vi "10-Tap 8-Bit Camera with DRAM (Host) - const.vi"() -> ()   [LabVIEW 2018]
doc: "This is the host VI for the 10-Tap 8-Bit Camera with DRAM example. This example demonstrates how to acquire images from a 10-tap, 8-bit, extended configuration, Camera Link camera and display the images on the host. This example supports area scan and line scan cameras for both continuous and finite acquisitions.\n\nThis example also demonstrates the use of DRAM as a frame buffer for very high speed acquisitions. Data packing and flow-control are also employed to maximize use of the available DRAM and FIFOs in terms of both memory space and performance.\n\nAdditionally, the example demonstrates the serial server, which allows third-party camera configuration utilities to communicate with the camera using the Camera Link serial interface while this VI is running."
uses:
  <vilib>/userdefined/High Color/nirio_resource_hc.ctl
  <vilib>/Analysis/Matrix/Datatypes/RealMatrix.ctl
  <vilib>/Platform/TimedLoop/XDataNode/timing_clust.ctl
  <vilib>/Platform/TimedLoop/XDataNode/nitl_modes.ctl
  <vilib>/Platform/TimedLoop/XDataNode/wakeup.ctl
  <vilib>/DAQmx/write.llb/DAQmx Write (Analog DBL 1Chan 1Samp).vi
  <vilib>/Analysis/baseanly.llb/Real A x B.vi
  <vilib>/FPGAPlugInAG/PCIe-1473R/niLvFpga_Open_PCIe-1473R.vi
  <vilib>/rvi/interface/common/dynamic/niFpgaDynamicAddResources.vi
  <vilib>/FPGAPlugInAG/Dynamic/niLvFpga_Reset_Dynamic.vi
  <vilib>/Analysis/Matrix/Numeric/Conversions/Array To Matrix - RA2.vi
  <userlib>/DAQNavi Polymorphic VI/create/DAQNavi Create Channel(CI-UpDown Count Value).vi
  <vilib>/Utility/error.llb/Error Cluster From Error Code.vi
  <vilib>/rvi/errors/niLvFpgaAdjustHostInterfaceError.vi
  <vilib>/FPGAPlugInAG/Dynamic/niLvFpga_Run_Dynamic.vi
  <vilib>/rvi/interface/common/niFpgaWaitOnOcc.vi
  <userlib>/DAQNavi Polymorphic VI/read/DAQNavi Read (Counter Count Value 1Chan 1Samp).vi
  <vilib>/Analysis/Matrix/Numeric/Conversions/Array To Matrix - RA.vi
  <vilib>/Analysis/Matrix/Numeric/Conversions/Matrix To Array - RM.vi
  <vilib>/DAQmx/miscellaneous.llb/DAQmx Fill In Error Info.vi
  <vilib>/FPGAPlugInAG/Dynamic/niLvFpga_Close_Dynamic.vi
  <vilib>/platform/TimedLoop/XDataNode/XDataNode.xnode
  <vilib>/rvi/interface/nirviOpenFPGA/nirviOpenFPGA.xnode
  FPGA Bitfiles/10-Tap8-bitCamer_FPGATarget_10-Tap8-bitCamer_C490DC32.lvbitx
  <vilib>/rvi/interface/nirviMethod/nirviMethod.xnode
  <vilib>/ErrorRing/Error Ring.xnode
  <vilib>/rvi/interface/nirviReadWriteControl/nirviReadWriteControl.xnode
  <vilib>/rvi/interface/nirviCloseFPGA/nirviCloseFPGA.xnode
  <vilib>/rvi/interface/Simulation/niFpgaSimulationCallBeginRW.vi
  <vilib>/rvi/errors/niLvFpgaMergeErrorWithErrorCode.vi
  NiFpgaLv.dll
  <vilib>/FPGAPlugInAG/Dynamic/niLvFpga_ConfigureFifo_Dynamic.vi
  <vilib>/FPGAPlugInAG/Dynamic/niLvFpga_StartFifo_Dynamic.vi
  <vilib>/FPGAPlugInAG/Dynamic/niLvFpga_ReadFifo_Dynamic.vi
  <vilib>/Platform/TimedLoop/XDataNode/XDNodeRunTimeDep.lvlib
  <resource>/objmgr/ni.dex.rc
  MPC_dll_4_vs17_cv3_4/x64/Release/MPC_dll_4_vs17_cv3_4.dll
  fish tracking dll vc17 opencv3_4/x64/Release/fish tracking dll vc17 opencv3_4.dll
  <vilib>/Analysis/NI_AALBase.lvlib
  <vilib>/Analysis/Matrix/NI_Matrix.lvlib
panel:
  in  "shift":i32=9
  in  "gamma":dbl=0.015 format="%#_13g"
  out "Cluster":cluster{"data":i32, i32}
  out "Real Matrix 5":T1
  out "Real Matrix 4":T1
  out "Real Matrix 2":T1
  out "Real Matrix":T1
  out "A x B 2":T1
  out "A x B":T1
  out "error out":errorcluster
  in  "send":bool
  out "Is Connected":bool
  in  "update ratio":dbl=0.1
  in  "Start Serial Server":bool=TRUE
  in  "Stopped 2":bool
  in  "display":bool=TRUE
  out "Image":T2(plugin-control)
  in  "reset 2":bool
  in  "reset frame":bool
  in  "reset position":bool
  out "max load a frame":dbl
  out "max load a position":dbl
  out "# elements in queue":i32
  out "element":dbl[](array[numeric])
  in  "start sending":bool
  out "connected":bool
  in  "Acquire":bool
  out "max distance 2":i32
  out "out of FOV 2":i32
  in  "count":bool
  out "max distance":i32
  out "out of FOV":i32
  out "Stage Position Y":i32=520
  out "Stage Position X":i32=520
  out "#timeout3":i32
  out "#timeout1":i32
  out "max time4 image and position loading":dbl
  out "max time3 total":dbl
  out "max time2 detection":dbl
  out "max time1 detection+command":dbl
  out "time loading a frame":dbl
  in  "length of fish_history":i32=4
  in  "m(length of kernel)":i32=30
  out "Heading":cluster{dbl, dbl}
  out "BKG_Global":T2(plugin-control)
  out "process":i32
  in  "Target Y":i32(slide)=171 min=0 max=384 scale=130.0..230.0
  in  "Target X":i32(slide)=179 min=0 max=520 scale=130.0..230.0
  out "y":dbl
  out "x":dbl
  in  "Controller":picture
  out "Y Resolution":i32
  out "X Resolution":i32
  in  "Track":bool
  out "Frame #":i32=72
  out "电压2":dbl
  out "电压1":dbl
  out "fish FOUND":bool
  out "Centroid":cluster{"x":i32, "y":i32}
  out "TimeDelay":dbl
  in  "DMA Buffer Size\n(In Images)":u32=64 caption="DMA Buffer Size"
  in  "Signal Mapping":T3(ring)=enum."Basler 10-tap"
  out "Acq In Progress":bool
  in  "Line Scan":bool
  in  "Cancel":bool
  out "Acq'd Frame Width":u32
  in  "Stopped":bool
  in  "RIO Device":T4="RIO0"
  out "DMA Write Timeout":bool
  out "Frames Acq'd":u32
  out "Acq'd Frame Height":u32
  in  "Stop":bool
  in  "Image Height":u32=360 max=65535
  in  "Image Width":u32=360 max=65535 step=40
  out "Initialized":bool
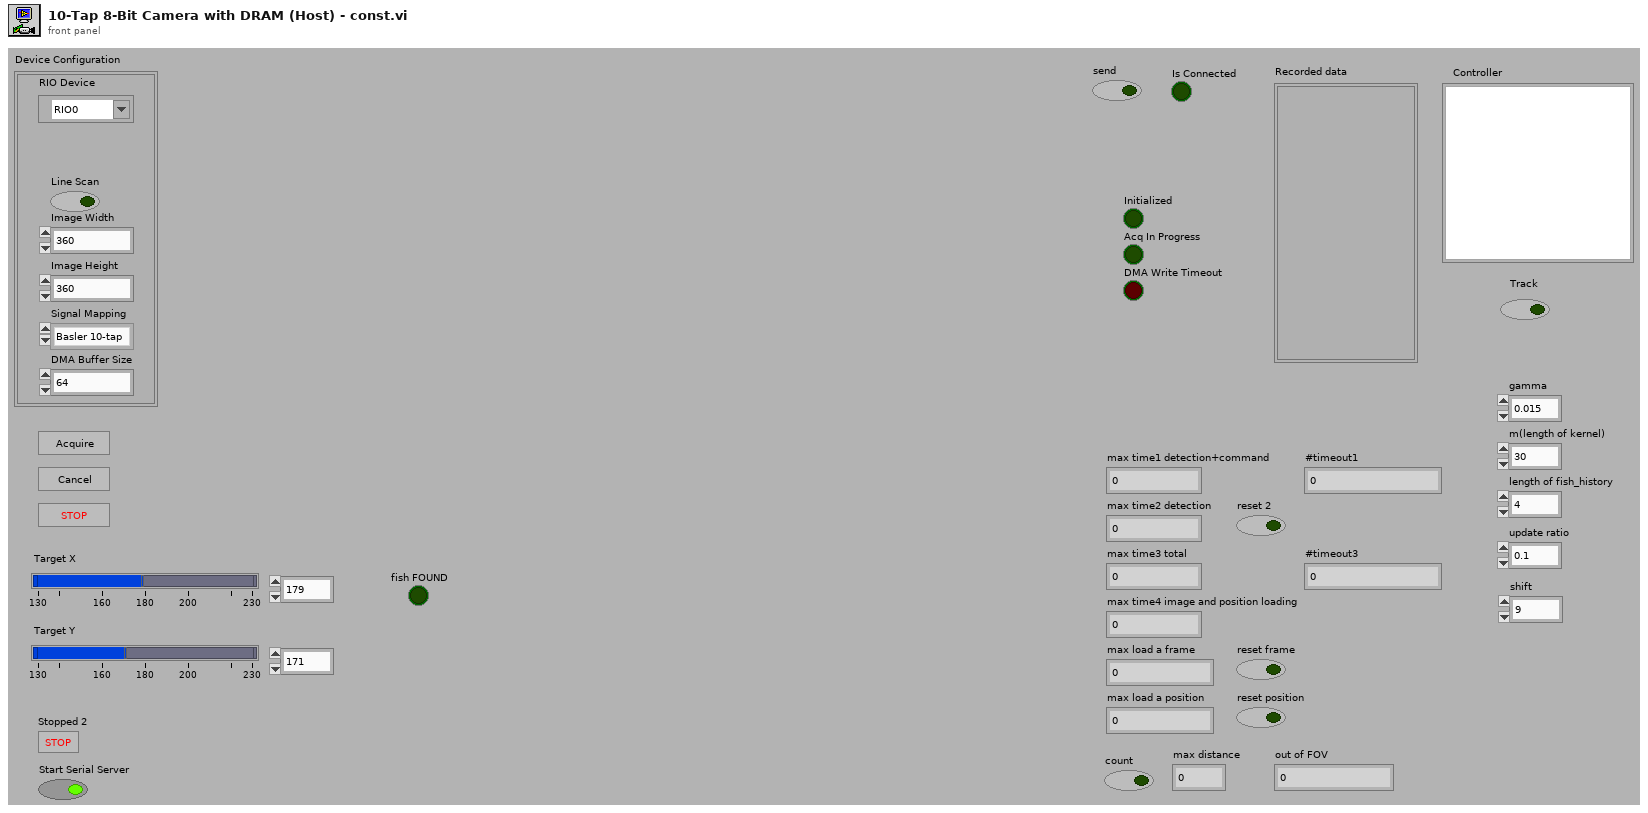
[diagram p1: front panel]
types:
  T1 = typedef "NI_Matrix.lvlib/RealMatrix.ctl" = dbl[][]
  T2 = typedef "IMAQ Image.ctl" = refnum<image>
  T3 = enum8{"Standard", "Basler 10-tap", "Vosskühler 10-tap"}
  T4 = typedef "nirio_resource_hc.ctl" = tag
  T5 = typedef "Image Type" = u32
  T6 = typedef "XDNodeRunTimeDep.lvlib/timing_clust.ctl" = cluster{"Expected End [f-1]":u64, "Actual End [f-1]":u64, "Finished Late? [f-1]":bool, "Expected End [i-1]":u64, "Actual End [i-1]":u64, "Finished Late? [i-1]":bool, "Expected Start [i]":u64, "Actual Start [i]":u64, "Expected Start [f]":u64, "Actual Start [f]":u64, "Source Name":string, "Structure Name":string, "Period":i64, "Deadline":i64, "Offset":i64, "Start":i64, "Priority":i32, "Timeout":i32, "Mode":T7, "Wakeup Reason":T8, "Error":errorcluster, "Source Type":string, "Secondary Source Type":string, "Global End Time":u64, "Global Start Time":u64, "Frame Duration":u64, "Iteration Duration":u64, "Assigned CPU":i32, "I/O Scan Engine Mode":u32}
  T7 = typedef "XDNodeRunTimeDep.lvlib/nitl_modes.ctl" = enum32{"No Change", "Process missed periods, maintain original phase", "Discard missed periods, maintain original phase", "Process missed periods, ignore original phase", "Discard missed periods, ignore original phase"}
  T8 = typedef "XDNodeRunTimeDep.lvlib/wakeup.ctl" = enum32{"Normal", "Aborted", "Asynchronous wakeup", "Timing source error", "Timed loop error", "Timeout"}
  T9 = enum16{"big-endian, network order", "native, host order", "little-endian"}
  T10 = enum32{"Map Pixel Pointer", "Unmap Pixel Pointer", "Get Pixels Infos"}
  T11 = typedef "LVPoint32TypeDef.ctl" = cluster{"Horizontal":i32, "Vertical":i32}
  T12 = typedef "LVPositionTypeDef.ctl" = cluster{"Left":i32, "Top":i32}
  T13 = typedef "LVBoundsTypeDef.ctl" = cluster{"Width":u32, "Height":u32}
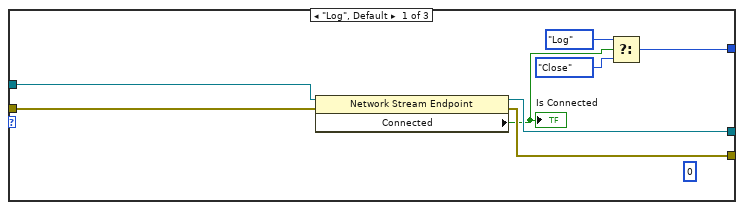
[diagram p4: hidden frame]
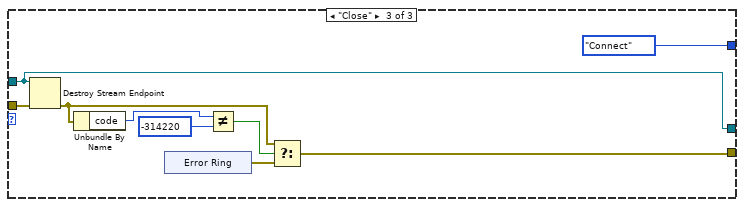
[diagram p5: hidden frame]
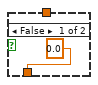
[diagram p12: hidden frame]
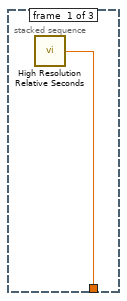
[diagram p13: hidden frame]
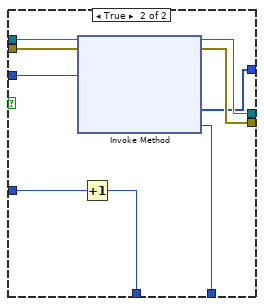
[diagram p14: hidden frame]
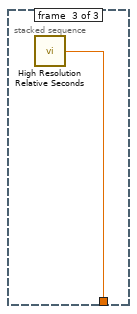
[diagram p15: hidden frame]
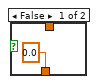
[diagram p16: hidden frame]
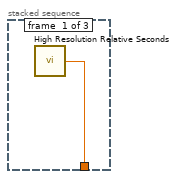
[diagram p17: hidden frame]
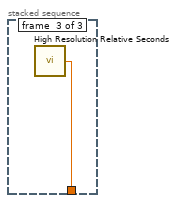
[diagram p20: hidden frame]
diagram:
  w23 = 72 ("n_templates")
  w25 = 0
  w46 = 2
  w40 = 0
  w47 = 0.0
  w72 = T5 0 items=["Grayscale (U8)", "Grayscale (I16)", "Grayscale (SGL)", "Complex (CSG)", "RGB (U32)", "HSL (U32)", "RGB (U64)", "Grayscale (U16)"] ("Image Type")
  w86 = refnum<k21> "Stage_Y"  # DAQmx任务名
  w87 = refnum<k21> "Stage_X"  # DAQmx任务名
  w89 = T5 0 items=["Grayscale (U8)", "Grayscale (I16)", "Grayscale (SGL)", "Complex (CSG)", "RGB (U32)", "HSL (U32)", "RGB (U64)", "Grayscale (U16)"] ("Image Type")
  w95 = u32 8  # Pixels per DMA word
  w126 = T5 0 items=["Grayscale (U8)", "Grayscale (I16)", "Grayscale (SGL)", "Complex (CSG)", "RGB (U32)", "HSL (U32)", "RGB (U64)", "Grayscale (U16)"] ("Image Type")
  # "Start the Serial Server to allow serial communication\nwith the camera. This allows third-party camera\nconfiguration utilites to be used."
  # "If your camera outputs active-low enable\nsignals or does not use DVAL then you \ncan change the configuration here."
  # "Configure the DMA FIFO memory buffer to be\nlarge enough for several frames. This provides\nbuffering to help deal with system latencies."
  # "Start running\nthe FPGA VI."
  # "Reset FPGA to clear\nany current state."
  # "Read the specified image\nwidth and height. In this\nexample, these must be set\nbefore starting the VI."
  # "Merge any errors.\nClean up the image.\nClose the FPGA reference.\nDisplay any errors."
  # "Acquire frames as requested.\nUse the width and height to determine how much data to read from the DMA FIFO.\nConvert the data into a Vision Image for display."
  # "Monitor the acquisition status"
  # "Create an image of the type to be displayed."
  # "Initialize the acquisition interface on the FPGA.  This will\nwait until a pixel clock is detected from the camera."
  # "Initialize the DMA FIFO for transferring\ndata from FPGA target to the host."
  # "Configure the Camera Link interface.\nThis needs to be done prior to running\nthe FPGA block diagram."
  # "Open a reference to the FPGA bitstream\nand initialize the user interface."
  n1 = flat-sequence {
    tunnel: [w132] -> w121
    tunnel: [w131] -> w130
    frame #0 {
      w135 = u32 0 ("Num Lines Acq'd")
      w134 = FALSE ("stop")
      n2 = local write "DMA Write Timeout"(w134) -> ()
      n3 = local write "Acq'd Frame Width"(w135) -> ()
      n4 = local write "Acq'd Frame Height"(w135) -> ()
      n5 = local write "Stopped"(w134) -> ()
      n6 = local write "Frames Acq'd"(w135) -> ()
      n7 = local write "Initialized"(w134) -> ()
      n8 = xnode "打开FPGA VI引用句柄"("resource name"="RIO Device") -> ("FPGA VI Reference Out"=w132:refnum<k20>, "error out"=w131:errorcluster)  [unwired: 1 in]
    }
  }
  n9 = xnode "Invoke Method"("FPGA VI Reference In"=w121, "error in"=w130) -> ("FPGA VI Reference Out"=w111:refnum<k20>, "error out"=w113:errorcluster)
  n10 = xnode "Read/Write Control"("FPGA VI Reference In"=w111, "error in"=w113, "CL Config.FVAL Active High"=TRUE ("IO Module Config.CL FVAL Active High"), "CL Config.LVAL Active High"=TRUE ("IO Module Config.CL LVAL Active High"), "CL Config.DVAL Active High"=TRUE ("IO Module Config.CL DVAL Active High"), "CL Config.Spare Active High"=TRUE ("IO Module Config.CL Spare Active High"), "CL Config.Line Scan"="Line Scan", "Acq Control.Ignore DVAL"=FALSE ("CL Config.Line Scan"), "CL Config.Configuration"=enum8{"Base", "Medium", "Full"}."Full", "CL Config.Signal Mapping"="Signal Mapping") -> ("FPGA VI Reference Out"=w114:refnum<k20>, "error out"=w112:errorcluster)
  n11 = xnode "Invoke Method"("FPGA VI Reference In"=w114, "error in"=w112) -> ("FPGA VI Reference Out"=w92:refnum<k20>, "error out"=w91:errorcluster)  [unwired: 1 in]
  n12 = Multiply(x="Image Height", y="Image Width") -> (x*y=w94:u32)
  n13 = Quotient & Remainder(x=w94, y=w95) -> (floor(x/y)=w93:u32)  [unwired: 1 out]
  n14 = Multiply(x=w93, y="DMA Buffer Size\n(In Images)") -> (x*y=w105:u32)
  n15 = xnode "Invoke Method"("FPGA VI Reference In"=w92, "error in"=w91, "请求的深度"=w105) -> ("FPGA VI Reference Out"=w120:refnum<k20>, "error out"=w119:errorcluster)  [unwired: 1 out]
  n16 = xnode "Invoke Method"("FPGA VI Reference In"=w120, "error in"=w119) -> ("FPGA VI Reference Out"=w106:refnum<k20>, "error out"=w118:errorcluster)
  n17 = xnode "读取/写入控件"("FPGA VI Reference In"=w106, "error in"=w118, "Acq Control.Initialize"=TRUE ("Arm Acquisition")) -> ("FPGA VI Reference Out"=w129:refnum<k20>, "error out"=w128:errorcluster)
  n18 = while {
    tunnel: w129 -> [w143]
    tunnel: w128 -> [w142]
    tunnel: [w141] -> w10
    tunnel: [w145] -> w102
    i -> [w137]
    stop <- w148 stop-if-true
    # "A custom error is generated if the acquisition unit has not become\ninitialized within 2 seconds. This typically occurs when a camera is\nnot connected, is not powered, or is not of the correct type."
    n19 = xnode "读取/写入控件"("FPGA VI Reference In"=w143, "error in"=w142) -> ("FPGA VI Reference Out"=w141:refnum<k20>, "error out"=w140:errorcluster, "Acq Status.Initialized"=w139:bool)
    n20 = Wait (ms)(milliseconds to wait=u32 100) -> ()  [unwired: 1 out]
    n21 = Greater?(x=w137, y=20) -> (0:w138:bool)
    n22 = case shown="True" w138 {
      tunnel: [w150 FALSE] -> w144
      tunnel: w139 -> [w150 _]
      tunnel: w140 -> [w149 w152]
      tunnel: [w149 w154] -> w145
      frame False {
      }
      frame True {
        n23 = Merge Errors(w152, errorcluster {"status"=TRUE, "code"=-8999, "source"="Acquisition Initialization: This error typically occurs when a camera is not properly connected, is not powered, or is not of the correct type."} ("error in")) -> (w154:errorcluster)
      }
    }
    "Initialized" <- w144
    n24 = Unbundle By Name(w145) -> ("status"=w147:bool)
    n25 = Or(x=w147, y=w144) -> (x .or. y?=w148:bool)
  }
  n26 = case shown="True" "Start Serial Server" {
    tunnel: [_ w155] -> w9
    tunnel: w10 -> [_ w156]
    frame False {
    }
    frame True {
      n27 = control-ref of="Stopped 2"() -> (w157:refnum<vi>)
      n28 = call "SerialServer.vi"("Stop Refnum"=w157, "FPGA VI Reference In"=w156) -> ("FPGA VI Reference Out"=w155:refnum<k20>)  [unwired: 5 in]
    }
  }
  n29 = call "IMAQ Create"("Image Name"="Image", "Image Type"=w126, "error in (no error)"=w102) -> ("New Image"=w99:T2, "error out"=w98:errorcluster)  [unwired: 2 in]
  n30 = Add(x="length of fish_history", y=1) -> (x+y=w42:i32)
  n31 = Initialize Array(0.0, 7) -> (w12:dbl[])
  n32 = Obtain Queue(max queue size (-1, unlimited)=3, name (unnamed)="tracking result" ("Image Name"), element data type=w12) -> (queue out=w8:refnum<queue>)  [unwired: 2 in, 2 out]
  n33 = Multiply(x=w46, y=w42) -> (x*y=w39:i32)
  n34 = To Unsigned Byte Integer(number=w25) -> (unsigned 8bit integer=w26:u8)
  n35 = Add(x="m(length of kernel)", y=1) -> (x+y=w27:i32)
  n36 = Initialize Array(w26, w25, w25, w25) -> (w24:u8[][][])
  n37 = for {
    N: w23 -> [_]
    shift-right: [w159] -> w22
    shift-left: w24 -> [w160]
    i -> [w158]
    w164 = T5 0 items=["Grayscale (U8)", "Grayscale (I16)", "Grayscale (SGL)", "Complex (CSG)", "RGB (U32)", "HSL (U32)", "RGB (U64)", "Grayscale (U16)"] ("Image Type")
    n38 = Number To Decimal String(number=w158) -> (decimal integer string=w168:string)  [unwired: 1 in]
    n39 = Concatenate Strings(w168, ".jpg") -> (w167:string)
    n40 = Build Path(base path=path "F:/TrackingUsingOpenCV3_with_bkg_subtr_and_pred_and_temp_matching_nodisplay - 210309/templates" ("Templates Path"), name or relative path=w167) -> (appended path=w166:path)
    n41 = call "IMAQ Create"("Image Name"="Temp", "Image Type"=w164) -> ("New Image"=w163:T2)  [unwired: 3 in, 1 out]
    n42 = call "IMAQ ReadFile"("File Path"=w166, "Image"=w163) -> ("Image Out"=w162:T2)  [unwired: 5 in, 4 out]
    n43 = call "IMAQ ImageToArray"("Image"=w162) -> ("Image Pixels (U8)"=w161:u8[][])  [unwired: 3 in, 4 out]
    n44 = Insert Into Array(array=w160, index (dim 0)=w158, new element=w161) -> (w159:u8[][][])  [unwired: 2 in]
  }
  n45 = Multiply(x=w46, y=w27) -> (x*y=w45:i32)
  n46 = Obtain Queue(max queue size (-1, unlimited)=w45, name (unnamed)="command_history", element data type=w47) -> (queue out=w49:refnum<queue>)  [unwired: 2 in, 2 out]
  n47 = Obtain Queue(max queue size (-1, unlimited)=w39, name (unnamed)="stage_position_history", element data type=w40) -> (queue out=w38:refnum<queue>)  [unwired: 2 in, 2 out]
  n48 = Obtain Queue(max queue size (-1, unlimited)=w39, name (unnamed)="fish_tr_history", element data type=w40) -> (queue out=w51:refnum<queue>)  [unwired: 2 in, 2 out]
  n49 = Obtain Queue(max queue size (-1, unlimited)=w39, name (unnamed)="fish_heading_history", element data type=w47) -> (queue out=w50:refnum<queue>)  [unwired: 2 in, 2 out]
  n50 = for "For循环" {
    N: w45 -> [_]
    tunnel: w49 -> [w173]
    tunnel: [w172] -> w48
    n51 = Lossy Enqueue Element(queue=w173, element=0.0) -> (queue out=w172:refnum<queue>)  [unwired: 1 in, 3 out]
  }
  n52 = call-poly <userlib>:"DAQNavi Create Channel.vi"("physical channels"="PCI-1784,BID#1/cntr0" ("Image Name"), "signal counting type"="AbPhaseX4" ("Image Name"), "initial value"="0" ("Image Name")) -> ("task out"=w66:i32)  [unwired: 11 in, 1 out]
  n53 = call-poly <userlib>:"DAQNavi Create Channel.vi"("physical channels"="PCI-1784,BID#1/cntr1" ("Image Name"), "signal counting type"="AbPhaseX4" ("Image Name"), "initial value"="0" ("Image Name")) -> ("task out"=w65:i32)  [unwired: 11 in, 1 out]
  n54 = call "IMAQ Create"("Image Name"="BkgImageOpenCV", "Image Type"=w72) -> ("New Image"=w74:T2)  [unwired: 3 in, 1 out]
  n55 = call <userlib>:"DAQNavi Start Task.vi"("task in"=w66) -> ("task out"=w62:i32)  [unwired: 9 in, 1 out]
  n56 = call <userlib>:"DAQNavi Start Task.vi"("task in"=w65) -> ("task out"=w61:i32)  [unwired: 9 in, 1 out]
  n57 = while "Target->Host Data Writer" {
    shift-right: [w181] -> w2
    shift-left: _ -> [w184]
    shift-right: [w180] -> _
    shift-left: _ -> [w185]
    shift-right: [w182] -> _
    shift-left: enum16{"Log", "Connect", "Close"}."Log" -> [w183]
    tunnel: w8 -> [w176]
    tunnel: [w175] -> w1
    stop <- w174 stop-if-true
    # "Send Data to Host VI"
    n58 = case shown="\"Connect\"" w183 {
      tunnel: [w202 w209 w227] -> w180
      tunnel: w185 -> [w205 _ w227]
      tunnel: w184 -> [w204 _ w228]
      tunnel: [w203 w210 w221] -> w181
      tunnel: [w206 enum16{"Log", "Connect", "Close"}."Log" enum16{"Log", "Connect", "Close"}."Connect"] -> w182
      frame "Log", Default {
        (unwired) 0 ("timeout ms")
        n59 = property class="Network Stream Endpoint"(reference=w205, error in=w204) -> (reference out=w202:refnum<k21>, error out=w203:errorcluster, "Connected"=w201:bool)
        "Is Connected" <- w201
        n60 = Select(t=enum16{"Log", "Connect", "Close"}."Log", s=w201, f=enum16{"Log", "Connect", "Close"}."Close") -> (s? t:f=w206:enum16{"Log", "Connect", "Close"})
      }
      frame "Connect" {
        n61 = Concatenate Strings("//" ("reader url"), "192.168.1.30" ("Target IP Address")) -> (w215:string)
        n62 = Concatenate Strings(w215, "/reader1" ("reader url")) -> (w213:string)
        n63 = Create Network Stream Writer Endpoint(5:-1 ("timeout in ms (-1)"), 7:70, 9:0.0, 10:w213, 11:"writer") -> (0:w210:errorcluster, 3:w209:refnum<k21>)  [unwired: 2 in]
      }
      frame "Close" {
        n64 = Destroy Stream Endpoint(8:w228, 11:w227) -> (0:w222:errorcluster)
        n65 = Unbundle By Name(w222) -> ("code"=w226:i32)
        n66 = xnode "Error Ring"() -> ("error out"=w223:errorcluster)
        n67 = Not Equal?(x=w226, y=-314220) -> (x != y?=w224:bool)
        n68 = Select(t=w222, s=w224, f=w223) -> (s? t:f=w221:errorcluster)
      }
    }
    n69 = property class="Network Stream Endpoint"(reference=w180, error in=w181) -> (reference out=w178:refnum<k21>, error out=w177:errorcluster, "Connected"=w179:bool)
    n70 = case shown="True" w179 {
      tunnel: w178 -> [_ w190]
      tunnel: w177 -> [_ w191]
      tunnel: w176 -> [w186 w189]
      tunnel: [w186 w187] -> w175
      frame False {
      }
      frame True {
        n71 = Get Queue Status(queue=w189) -> (queue out=w193:refnum<queue>)  [unwired: 2 in, 7 out]
        n72 = Dequeue Element(queue=w193) -> (queue out=w187:refnum<queue>, element=w192:dbl[])  [unwired: 2 in, 2 out]
        n73 = case shown="True" "send" {
          tunnel: w192 -> [_ w198]
          tunnel: w191 -> [_ w197]
          tunnel: w190 -> [_ w196]
          frame False {
          }
          frame True {
            w199 = 0 ("timeout ms (-1)")
            n74 = shared-variable-write(w196, w197, w198, w199) -> (w195:refnum<k21>, w200:errorcluster)  [unwired: 1 out]
            n75 = Flush Stream(8:w200, 9:w199, 11:w195) -> (0:→"error out":errorcluster)  [unwired: 1 in, 2 out]
          }
        }
      }
    }
    n76 = local read "Stop"() -> (w174:bool)
  }
  n77 = disable-structure shown="Disabled" {
    disable-tunnel: w8 -> [w231 _]
    frame Disabled {
      n78 = Concatenate Strings("//" ("reader url"), "192.168.1.19" ("Target IP Address")) -> (w242:string)
      n79 = Concatenate Strings(w242, "/reader1" ("reader url")) -> (w240:string)
      n80 = Create Network Stream Writer Endpoint(7:70, 9:0.0, 10:w240, 11:"writer") -> (0:w245:errorcluster, 3:w247:refnum<k21>)  [unwired: 3 in]
      n81 = property class="Network Stream Endpoint"(reference=w247, error in=w245) -> (reference out=w238:refnum<k21>, error out=w237:errorcluster, "Connected"=→"connected":bool)
      n82 = node-c288() -> (w251:T6)  [unwired: 4 in]
      n83 = timed-loop {
        tunnel: w231 -> [w258]
        tunnel: w238 -> [w257]
        tunnel: w237 -> [w256]
        tunnel: [w255] -> w234
        tunnel: [w254] -> w233
        tunnel: [w253] -> w232
        timing: w251 -> [_]
        timing-out: [_] -> w250
        stop <- w252 stop-if-true
        n84 = node-c288() -> ()  [unwired: 1 in, 1 out]
        n85 = case shown="True" "start sending" {
          tunnel: w257 -> [w263 w276]
          tunnel: w256 -> [w262 w275]
          tunnel: w258 -> [w264 w266]
          tunnel: [w264 w274] -> w255
          tunnel: [w263 w269] -> w254
          tunnel: [w262 w268] -> w253
          frame False {
          }
          frame True {
            w270 = 0
            n86 = Get Queue Status(queue=w266) -> (queue out=w267:refnum<queue>, # elements in queue=w265:i32)  [unwired: 2 in, 6 out]
            n87 = disable-structure shown="Disabled" {
              disable-tunnel: w265 -> [w277 _]
              frame Disabled {
                "# elements in queue" <- w277
              }
              frame Enabled {
              }
            }
            n88 = Dequeue Element(queue=w267) -> (queue out=w274:refnum<queue>, element=w273:dbl[])  [unwired: 2 in, 2 out]
            n89 = disable-structure shown="Disabled" {
              disable-tunnel: w273 -> [w278 _]
              frame Disabled {
                "element" <- w278
              }
              frame Enabled {
              }
            }
            n90 = shared-variable-write(w276, w275, w273, w270) -> (w272:refnum<k21>, w271:errorcluster)  [unwired: 1 out]
            n91 = Flush Stream(8:w271, 9:w270, 11:w272) -> (0:w268:errorcluster, 3:w269:refnum<k21>)  [unwired: 1 in, 1 out]
          }
        }
        n92 = local read "Stop"() -> (w252:bool)
        n93 = node-c288() -> ()  [unwired: 1 in, 1 out]
      }
      n94 = node-c288(w250) -> ()  [unwired: 1 out]
      n95 = Release Queue(queue=w234) -> ()  [unwired: 2 in, 3 out]
      n96 = Flush Stream(8:w232, 11:w233) -> (0:w235:errorcluster, 3:w236:refnum<k21>)  [unwired: 2 in, 1 out]
      n97 = Destroy Stream Endpoint(8:w235, 11:w236) -> ()  [unwired: 1 out]
    }
    frame Enabled {
    }
  }
  n98 = call-poly <vilib>:"Array To Matrix.vi"("Real 2D Array"=dbl[][] [[1.506559, -0.036078], [0.030048, 1.495542]]) -> ("Real Matrix"=w4:T1)
  "Real Matrix 5" <- w4
  n99 = call "IMAQ ReadFile"("File Path"=path "F:/TrackingUsingOpenCV3_with_bkg_subtr_and_pred_and_temp_matching_nodisplay/fish tracking dll vc17 opencv3_4/bkg_global.png" ("Bkg Image Path"), "Image"=w74) -> ("Image Out"=w71:T2)  [unwired: 5 in, 4 out]
  n100 = call-poly <vilib>:"Array To Matrix.vi"("Real 2D Array"=dbl[][] [[1.506559, -0.036078, 0.0], [0.030048, 1.495542, 1.506559], [-12.463135, -1.547689, 1.0]]) -> ("Real Matrix"=w5:T1)
  "Real Matrix 4" <- w5
  n101 = node-c288() -> (w17:T6)  [unwired: 4 in]
  n102 = call "IMAQ Create"("Image Name"="DstImageOpenCV", "Image Type"=w89) -> ("New Image"=w88:T2)  [unwired: 3 in, 1 out]
  n103 = while {
    tunnel: w10 -> [w291]
    tunnel: [w294] -> w115
    stop <- w293 stop-if-true
    w284 = u32 10  # Pixels per clock
    # "Update status indicators"
    n104 = Wait Until Next ms Multiple(millisecond multiple=u32 100) -> ()  [unwired: 1 out]
    n105 = xnode "Read/Write Control"("FPGA VI Reference In"=w291) -> ("error out"=w290:errorcluster, "Acq Status.Lines Per Frame"=w287:u32, "Acq Status.Frames Acq'd"=w289:u32, "Acq Status.Clocks Per Line"=w285:u32, "Acq Status.Acq In Progress"=→"Acq In Progress":bool, "Acq Status.DMA Write Timeout"=w282:bool)  [unwired: 1 in, 1 out]
    "DMA Write Timeout" <- w282
    n106 = Multiply(x=w285, y=w284) -> (x*y=w286:u32)
    n107 = disable-structure shown="Disabled" {
      disable-tunnel: w289 -> [w297 _]
      disable-tunnel: w287 -> [w296 _]
      disable-tunnel: w286 -> [w295 _]
      frame Disabled {
        "Acq'd Frame Height" <- w296
        "Frames Acq'd" <- w297
        "Acq'd Frame Width" <- w295
      }
      frame Enabled {
      }
    }
    n108 = local read "Stopped"() -> (w281:bool)
    n109 = Compound Arithmetic op=AND(w282, invert w281) -> (w283:bool)
    n110 = case shown="True" w283 {
      tunnel: w290 -> [w302 _]
      tunnel: [w302 errorcluster {"status"=TRUE, "code"=-8999, "source"="DMA Write Timeout: The write operation to the DMA FIFO on the FPGA timed out. This can be caused by the DMA FIFO not being started or the DMA FIFO overflowing. Make sure that Start is being called on the DMA FIFO. Also make sure that the host application is reading from the DMA FIFO fast enough to prevent it from overflowing."} ("error out")] -> w294
      frame False {
      }
      frame True {
      }
    }
    n111 = flat-sequence {
      tunnel: w294 -> [w301]
      tunnel: [w299] -> w293
      frame #0 {
        n112 = Unbundle By Name(w301) -> ("status"=w300:bool)
        n113 = Or(x=w300, y="Stopped") -> (x .or. y?=w299:bool)
        n114 = local write "Stopped"(w299) -> ()
      }
    }
  }
  n115 = call <vilib>:"Simple Error Handler.vi"("error in (no error)"=w2) -> ()  [unwired: 4 in, 5 out]
  n116 = Release Queue(queue=w1) -> ()  [unwired: 2 in, 3 out]
  n117 = Open/Create/Replace File(file path (use dialog)=path "E:/Time.txt" ("Folder"), operation (0:open)=4) -> (refnum out=w31:refnum<file>)  [unwired: 4 in, 2 out]
  n118 = call <vilib>:"DAQmx Start Task.vi"("task/channels in"=w86) -> ("task out"=w84:refnum<k21>)  [unwired: 13 in, 1 out]
  n119 = call <vilib>:"DAQmx Start Task.vi"("task/channels in"=w87) -> ("task out"=w85:refnum<k21>)  [unwired: 13 in, 1 out]
  n120 = timed-loop {
    tunnel: w10 -> [w427]
    tunnel: w98 -> [w426]
    tunnel: w93 -> [w323]
    tunnel: "Image Height" -> [w322]
    tunnel: "Image Width" -> [w431]
    tunnel: w99 -> [w430]
    tunnel: [w312] -> w116
    tunnel: [w429] -> w125
    tunnel: [w428] -> w123
    tunnel: w88 -> [w425]
    tunnel: w85 -> [w424]
    tunnel: w84 -> [w423]
    tunnel: [w422] -> w83
    tunnel: [w421] -> w82
    tunnel: w71 -> [w420]
    tunnel: w62 -> [w413]
    tunnel: w61 -> [w412]
    tunnel: [w411] -> w58
    tunnel: [w410] -> w57
    shift-right: [w416] -> _
    shift-left: u32 0 -> [w417]
    shift-right: [w414] -> _
    shift-left: cluster{"y":i32, "x":i32} {"y"=0, "x"=0} ("Centroid") -> [w415]
    tunnel: w48 -> [w409]
    tunnel: w51 -> [w408]
    tunnel: w50 -> [w407]
    tunnel: w38 -> [w406]
    tunnel: [w405] -> w37
    tunnel: [w404] -> w36
    tunnel: [w403] -> w35
    tunnel: [w402] -> w34
    tunnel: w31 -> [w400]
    tunnel: [w399] -> w30
    shift-right: [w398] -> _
    shift-left: _ -> [w397]
    tunnel: w23 -> [w396]
    tunnel: w22 -> [w395]
    tunnel: w8 -> [w394]
    timing: w17 -> [_]
    timing-out: [_] -> w16
    border: u32 0 -> [_]
    tunnel: w5 -> [w308]
    tunnel: w4 -> [w306]
    i -> [w401]
    stop <- w418 stop-if-true
    # "Read one frame\nfrom DMA FIFO"
    # "If we're in an acquisition, wait until\nwe have at least one frame to read."
    n121 = node-c288() -> ()  [unwired: 1 in, 1 out]
    n122 = stacked-sequence {
      tunnel: [_ w442 _] -> w429
      tunnel: w427 -> [_ w441 _]
      tunnel: w426 -> [_ w440 _]
      tunnel: [_ w439 _] -> w312
      tunnel: [_ w438 _] -> w393
      tunnel: w323 -> [_ w437 _]
      tunnel: w322 -> [_ w436 _]
      tunnel: [w435 _ _] -> w320
      tunnel: [_ _ w490] -> w321
      frame #0 {
        n123 = call <vilib>:"High Resolution Relative Seconds.vi"() -> ("relative seconds"=w435:dbl)
      }
      frame #1 {
        n124 = while {
          tunnel: [w448] -> w438
          tunnel: w437 -> [w445]
          shift-right: [w456] -> w442
          shift-left: w441 -> [w455]
          shift-right: [w449] -> w439
          shift-left: w440 -> [w454]
          tunnel: w436 -> [w443]
          stop <- w444 stop-if-true
          n125 = feedback #1() -> (w450:u32)
          n126 = while {
            tunnel: w455 -> [w486]
            tunnel: w454 -> [w485]
            tunnel: [w483] -> w453
            tunnel: [w484] -> w452
            tunnel: w450 -> [w489]
            tunnel: [w487] -> w446
            stop <- w488 stop-if-true
            n127 = xnode "Read/Write Control"("FPGA VI Reference In"=w486, "error in"=w485, "Acq Control.Cancel Acq"="Cancel") -> ("FPGA VI Reference Out"=w484:refnum<k20>, "error out"=w483:errorcluster, "Acq Status.Acq In Progress"=w482:bool, "Acq Status.Frames Acq'd"=w481:u32)
            n128 = Greater?(x=w481, y=w489) -> (0:w487:bool)
            n129 = Compound Arithmetic op=OR(invert w482, w487) -> (w488:bool)
          }
          n130 = case shown="False" w446 {
            tunnel: w445 -> [w468 w479]
            tunnel: [w463 w478] -> w456
            tunnel: w453 -> [w470 w477]
            tunnel: w452 -> [w469 w476]
            tunnel: [w457 w475] -> w451
            tunnel: w450 -> [w458 w474]
            tunnel: [w462 w473] -> w449
            tunnel: [_ w472] -> w448
            tunnel: [w468 w471] -> w447
            tunnel: w443 -> [w467 _]
            frame False {
              n131 = xnode "Read/Write Control"("FPGA VI Reference In"=w469, "error in"=w470, "Acq Control.Line Scan Height"=w467, "Acq Control.Frames To Acq"=u32 0 ("Frames To Acquire")) -> ("FPGA VI Reference Out"=w465:refnum<k20>, "error out"=w464:errorcluster)
              n132 = call "Rising Edge Detect.vi"("Input"="Acquire") -> ("Pulse"=w461:bool)  [unwired: 4 in]
              n133 = xnode "Read/Write Control"("FPGA VI Reference In"=w465, "error in"=w464, "Acq Control.Acquire"=w461) -> ("FPGA VI Reference Out"=w463:refnum<k20>, "error out"=w462:errorcluster)
              n134 = Select(t=u32 0, s="Acquire", f=w458) -> (s? t:f=w457:u32)
            }
            frame True {
              n135 = xnode "Invoke Method"("FPGA VI Reference In"=w476, "error in"=w477, "元素数量"=w479) -> ("FPGA VI Reference Out"=w478:refnum<k20>, "error out"=w473:errorcluster, "数据"=w472:u64[], "剩余元素"=w471:u32)  [unwired: 1 in]
              n136 = Increment(x=w474) -> (x+1=w475:u32)
            }
          }
          n137 = feedback-in #1(w451) -> ()
          n138 = Less?(x=w447, y=w445) -> (x < y?=w444:bool)
        }
      }
      frame #2 {
        n139 = call <vilib>:"High Resolution Relative Seconds.vi"() -> ("relative seconds"=w490:dbl)
      }
    }
    n140 = disable-structure shown="Disabled" {
      disable-tunnel: w401 -> [w432 _]
      frame Disabled {
        "process" <- w432
      }
      frame Enabled {
      }
    }
    n141 = Not(x="reset frame") -> (.not. x?=w311:bool)
    n142 = Boolean To (0,1)(Boolean=w311) -> (0, 1=w316:i16)
    n143 = Subtract(x=w321, y=w320) -> (x-y=w317:dbl)
    n144 = feedback #2(-inf) -> (w319:dbl)
    n145 = Max & Min(x=w317, y=w319) -> (max(x,y)=w314:dbl)  [unwired: 1 out]
    n146 = Multiply(x=w314, y=w316) -> (x*y=w313:dbl)
    n147 = feedback-in #2(w313) -> ()
    n148 = case shown="True" w311 {
      tunnel: w314 -> [_ w434]
      tunnel: [0.0 w434] -> w310
      frame False {
      }
      frame True {
      }
    }
    "max load a frame" <- w310
    n149 = flat-sequence {
      tunnel: w397 -> [w512]
      tunnel: w406 -> [w513]
      tunnel: w407 -> [w514]
      tunnel: w408 -> [w515]
      tunnel: w409 -> [w516]
      tunnel: w412 -> [w510]
      tunnel: w413 -> [w511]
      tunnel: w415 -> [w517]
      tunnel: w417 -> [w518]
      tunnel: w420 -> [w519]
      tunnel: w425 -> [w520]
      tunnel: w393 -> [w521]
      tunnel: w430 -> [w522]
      tunnel: w431 -> [w523]
      tunnel: w322 -> [w524]
      tunnel: [w524] -> w392
      tunnel: [w523] -> w391
      tunnel: [w522] -> w390
      tunnel: [w521] -> w389
      tunnel: [w520] -> w388
      tunnel: [w519] -> w387
      tunnel: [w518] -> w386
      tunnel: [w517] -> w385
      tunnel: [w516] -> w384
      tunnel: [w515] -> w383
      tunnel: [w514] -> w382
      tunnel: [w513] -> w381
      tunnel: [w512] -> w380
      tunnel: [w509] -> w379
      tunnel: [w508] -> w378
      tunnel: [w507] -> w377
      tunnel: [w506] -> w376
      tunnel: w396 -> [w506]
      tunnel: [w505] -> w375
      tunnel: w395 -> [w505]
      tunnel: w394 -> [w504]
      tunnel: [w504] -> w374
      tunnel: w308 -> [w492]
      tunnel: [w492] -> w307
      tunnel: w306 -> [w491]
      tunnel: [w491] -> w304
      tunnel: [w571] -> w373
      tunnel: [w570] -> w372
      tunnel: [w569] -> w371
      tunnel: [w568] -> w370
      tunnel: [w567] -> w369
      tunnel: [w566] -> w368
      tunnel: [w565] -> w367
      tunnel: [w564] -> w366
      tunnel: [w546] -> w365
      tunnel: [w544] -> w364
      tunnel: [w563] -> w363
      tunnel: [w562] -> w362
      tunnel: [w561] -> w361
      tunnel: [w560] -> w360
      tunnel: [w556] -> w359
      tunnel: [w545] -> w358
      tunnel: w392 -> [w571]
      tunnel: w391 -> [w570]
      tunnel: w390 -> [w569]
      tunnel: w389 -> [w568]
      tunnel: w388 -> [w567]
      tunnel: w387 -> [w566]
      tunnel: w386 -> [w565]
      tunnel: w385 -> [w564]
      tunnel: w384 -> [w563]
      tunnel: w383 -> [w562]
      tunnel: w382 -> [w561]
      tunnel: w381 -> [w560]
      tunnel: w380 -> [w554]
      tunnel: w379 -> [w546]
      tunnel: w378 -> [w545]
      tunnel: w377 -> [w544]
      tunnel: [w543] -> w357
      tunnel: w376 -> [w543]
      tunnel: [w542] -> w356
      tunnel: w375 -> [w542]
      tunnel: [w541] -> w355
      tunnel: w374 -> [w541]
      tunnel: [w540] -> w309
      tunnel: w307 -> [w540]
      tunnel: [w539] -> w305
      tunnel: w304 -> [w539]
      tunnel: w401 -> [w623]
      tunnel: w400 -> [w622]
      tunnel: [w621] -> w399
      tunnel: w373 -> [w672]
      tunnel: w372 -> [w671]
      tunnel: w371 -> [w670]
      tunnel: w370 -> [w668]
      tunnel: w369 -> [w597]
      tunnel: w368 -> [w643]
      tunnel: w367 -> [w640]
      tunnel: w366 -> [w595]
      tunnel: w365 -> [w616]
      tunnel: w364 -> [w615]
      tunnel: w363 -> [w634]
      tunnel: w362 -> [w633]
      tunnel: w361 -> [w632]
      tunnel: w360 -> [w631]
      tunnel: w359 -> [w619]
      tunnel: [w598] -> w354
      tunnel: [w639] -> w353
      tunnel: [w616] -> w352
      tunnel: [w615] -> w351
      tunnel: [w603] -> w350
      tunnel: [w630] -> w349
      tunnel: [w629] -> w348
      tunnel: [w628] -> w347
      tunnel: [w627] -> w346
      tunnel: [w618] -> w345
      tunnel: [w617] -> w344
      tunnel: w358 -> [w604]
      tunnel: w357 -> [w613]
      tunnel: w356 -> [w611]
      tunnel: w355 -> [w606]
      tunnel: w309 -> [w584]
      tunnel: w305 -> [w583]
      tunnel: w354 -> [w918]
      tunnel: [w918] -> w343
      tunnel: w353 -> [w917]
      tunnel: [w917] -> w342
      tunnel: w352 -> [w916]
      tunnel: [w916] -> w341
      tunnel: w351 -> [w915]
      tunnel: [w915] -> w340
      tunnel: w350 -> [w914]
      tunnel: [w914] -> w339
      tunnel: w349 -> [w913]
      tunnel: [w913] -> w338
      tunnel: w348 -> [w912]
      tunnel: [w912] -> w337
      tunnel: w347 -> [w911]
      tunnel: [w911] -> w336
      tunnel: w346 -> [w910]
      tunnel: [w910] -> w335
      tunnel: w345 -> [w909]
      tunnel: [w909] -> w334
      tunnel: w344 -> [w908]
      tunnel: [w908] -> w333
      tunnel: w343 -> [w934]
      tunnel: w342 -> [w933]
      tunnel: w341 -> [w932]
      tunnel: w340 -> [w931]
      tunnel: w339 -> [w930]
      tunnel: w338 -> [w929]
      tunnel: w337 -> [w928]
      tunnel: w336 -> [w927]
      tunnel: w335 -> [w926]
      tunnel: [w925] -> w421
      tunnel: [w924] -> w422
      tunnel: w424 -> [w923]
      tunnel: w423 -> [w922]
      tunnel: w334 -> [w921]
      tunnel: w333 -> [w920]
      tunnel: [w934] -> w332
      tunnel: [w933] -> w331
      tunnel: [w932] -> w330
      tunnel: [w931] -> w329
      tunnel: [w930] -> w328
      tunnel: [w929] -> w327
      tunnel: [w928] -> w326
      tunnel: [w927] -> w325
      tunnel: [w926] -> w324
      tunnel: [w936] -> w402
      tunnel: [w937] -> w403
      tunnel: [w938] -> w404
      tunnel: [w939] -> w405
      tunnel: [w940] -> w414
      tunnel: [w941] -> w410
      tunnel: [w942] -> w411
      tunnel: [w943] -> w416
      tunnel: [w944] -> w428
      tunnel: w332 -> [w944]
      tunnel: w331 -> [w943]
      tunnel: w330 -> [w942]
      tunnel: w329 -> [w941]
      tunnel: w328 -> [w940]
      tunnel: w327 -> [w939]
      tunnel: w326 -> [w938]
      tunnel: w325 -> [w937]
      tunnel: w324 -> [w936]
      tunnel: [w935] -> w398
      frame #0 {
        n150 = stacked-sequence {
          tunnel: w511 -> [_ w534 _]
          tunnel: w510 -> [_ w533 _]
          tunnel: [_ w532 _] -> w509
          tunnel: [_ w531 _] -> w508
          tunnel: [_ w530 _] -> w507
          tunnel: [w527 _ _] -> w503
          tunnel: [_ _ w538] -> w502
          frame #0 {
            n151 = call <vilib>:"High Resolution Relative Seconds.vi"() -> ("relative seconds"=w527:dbl)
          }
          frame #1 {
            n152 = call-poly <userlib>:"DAQNavi Read.vi"("task in"=w533) -> ("data"=w529:i32, "task out"=w530:i32)  [unwired: 9 in]
            n153 = call-poly <userlib>:"DAQNavi Read.vi"("task in"=w534) -> ("data"=w535:i32, "task out"=w532:i32)  [unwired: 9 in]
            n154 = disable-structure shown="Disabled" {
              disable-tunnel: w535 -> [w537 _]
              frame Disabled {
                "Stage Position X" <- w537
              }
              frame Enabled {
              }
            }
            n155 = Negate(x=w529) -> (-x=w528:i32)
            n156 = disable-structure shown="Disabled" {
              disable-tunnel: w528 -> [w536 _]
              frame Disabled {
                "Stage Position Y" <- w536
              }
              frame Enabled {
              }
            }
            n157 = Bundle("data"=w535, w528) -> (w531:cluster{"data":i32, i32})  [unwired: 1 in]
          }
          frame #2 {
            n158 = call <vilib>:"High Resolution Relative Seconds.vi"() -> ("relative seconds"=w538:dbl)
          }
        }
        n159 = Not(x="reset position") -> (.not. x?=w495:bool)
        n160 = Boolean To (0,1)(Boolean=w495) -> (0, 1=w497:i16)
        n161 = Subtract(x=w502, y=w503) -> (x-y=w499:dbl)
        n162 = feedback #3(-inf) -> (w501:dbl)
        n163 = Max & Min(x=w499, y=w501) -> (max(x,y)=w494:dbl)  [unwired: 1 out]
        n164 = Multiply(x=w494, y=w497) -> (x*y=w496:dbl)
        n165 = feedback-in #3(w496) -> ()
        n166 = case shown="True" w495 {
          tunnel: w494 -> [_ w526]
          tunnel: [0.0 w526] -> w493
          frame False {
          }
          frame True {
          }
        }
        "max load a position" <- w493
      }
      frame #1 {
        n167 = call <vilib>:"High Resolution Relative Seconds.vi"() -> ("relative seconds"=w556:dbl)
        n168 = feedback #4() -> (w557:dbl)  [unwired: 1 in]
        n169 = feedback-in #4(w556) -> ()
        n170 = Subtract(x=w556, y=w557) -> (x-y=w559:dbl)
        "TimeDelay" <- w559
        n171 = Greater?(x=w559, y=0.0045) -> (0:w551:bool)
        n172 = Subtract(x=w556, y=w554) -> (x-y=→"time loading a frame":dbl)
        n173 = Select(t=1, s=w551, f=0) -> (s? t:f=w548:i32)
        n174 = feedback #5(0) -> (w549:i32)
        n175 = Add(x=w548, y=w549) -> (x+y=w547:i32)
        "#timeout3" <- w547
        n176 = feedback-in #5(w547) -> ()
      }
      frame #2 {
        w650 = 30.0 ("pixel/mm")
        w635 = 0.0
        w653 = T10."Map Pixel Pointer" ("Function")
        # "Convert U64 array\nto U8 array"
        # "Convert array to\nimage for display"
        n177 = disable-structure shown="Disabled" {
          disable-tunnel: w643 -> [w684 _]
          frame Disabled {
            "BKG_Global" <- w684
          }
          frame Enabled {
          }
        }
        n178 = Add(x=1, y=w640) -> (x+y=w639:u32)
        n179 = Flatten To String(anything=w668, prepend array or string size? (T)=FALSE, byte order (0:big-endian, network order)=T9."native, host order") -> (data string=w666:string)  [unwired: 1 in, 2 out]
        n180 = disable-structure shown="Disabled" {
          disable-tunnel: w639 -> [w674 _]
          frame Disabled {
            "Frame #" <- w674
          }
          frame Enabled {
          }
        }
        n181 = String To Byte Array(string=w666) -> (unsigned byte array=w665:u8[])
        n182 = call "IMAQ GetImageSize"("Image"=w643) -> ("Y Resolution"=w641:i32, "X Resolution"=w642:i32)  [unwired: 3 in, 1 out]
        n183 = Reshape Array(w665, w672, w671) -> (w669:u8[][])
        n184 = call "IMAQ ArrayToImage"("Image Pixels (U8)"=w669, "Image"=w670) -> ("Image Out"=w598:T2)  [unwired: 8 in, 1 out]
        n185 = call "IMAQ GetImagePixelPtr"("Function"=w653, "Image"=w643) -> ("LineWidth(Pixels)"=w655:i32, "Pixel Pointer out"=w656:u64)  [unwired: 4 in, 4 out]
        n186 = expression code="atan(x)"(-0.043 ("tan(theta)")) -> (w644:dbl)
        n187 = Divide(x=w650, y=10000.0) -> (x/y=w647:dbl)
        n188 = Divide(x=w650, y=12800.0) -> (x/y=w646:dbl)
        n189 = call "IMAQ GetImageSize"("Image"=w598) -> ("Y Resolution"=w607:i32, "X Resolution"=w608:i32)  [unwired: 3 in, 1 out]
        "X Resolution" <- w608
        "Y Resolution" <- w607
        n190 = call "IMAQ GetImagePixelPtr"("Function"=w653, "Image"=w598) -> ("LineWidth(Pixels)"=w660:i32, "Pixel Pointer out"=w664:u64)  [unwired: 4 in, 4 out]
        n191 = disable-structure shown="Disabled" {
          disable-tunnel: w604 -> [w673 _]
          frame Disabled {
            "Cluster" <- w673
          }
          frame Enabled {
          }
        }
        n192 = call "IMAQ SetImageSize"("Y Resolution"=w607, "X Resolution"=w608, "Image"=w597) -> ("Image Out"=w605:T2)  [unwired: 2 in, 1 out]
        n193 = Bundle(w635, w635) -> (w610:cluster{dbl, dbl})  [unwired: 1 in]
        n194 = call "IMAQ GetImagePixelPtr"("Function"=w653, "Image"=w605) -> ("LineWidth(Pixels)"=w662:i32, "Pixel Pointer out"=w663:u64)  [unwired: 4 in, 4 out]
        n195 = dll-call lib="F:/TrackingUsingOpenCV3_with_bkg_subtr_and_pred_and_temp_matching_nodisplay - 210309/fish tracking dll vc17 opencv3_4/x64/Release/fish tracking dll vc17 opencv3_4.dll" fn="?find_centroid@@YAHPEADH0H0HHHHHPEAEHHPEAV?$Point_@H@cv@@NNNHHHHHHH22PEAV?$Point_@N@2@N@Z"("ImagePtrSrc"=w664, "LineWidthSrc"=w660, "ImagePtrDst"=w663, "LineWidthDst"=w662, "ImagePtrBkg"=w656, "LineWidthBkg"=w655, "Width"=w608, "Height"=w607, "BkgWidth"=w642, "BkgHeight"=w641, "templates"=w611, "n_templates"=w613, "TemplatesSize"=48 ("Templates size"), "position"=w604, "scale_x"=w647, "scale_y"=w646, "theta"=w644, "BinThreshold"=80, "counting_threshold"=200 ("Object Threshold"), "ROI_witdth"=110, "ROI_height"=110, "width_fish"=20, "length_fish"=115, "shift"="shift", "centroid_in"=w595, "centroid_out"=w595, "heading_vector"=w610, "Update_Ratio_Bkg"="update ratio") -> ("return type"=w638:i32, "centroid_out"=w603:cluster{"y":i32, "x":i32}, "heading_vector"=w602:cluster{dbl, dbl})  [unwired: 29 in, 2 out]
        "Centroid" <- w603
        "Heading" <- w602
        n196 = Quotient & Remainder(x=w623, y=2) -> (x-y*floor(x/y)=w625:i32)  [unwired: 1 out]
        n197 = Equal To 0?(x=w638) -> (x = 0?=w609:bool)
        "fish FOUND" <- w609
        n198 = Equal?(x=w625, y=0) -> (x = y?=w593:bool)
        n199 = Unbundle(w604) -> ("data"=w601:i32, w600:i32)
        n200 = Unbundle(w602) -> (w576:dbl, w575:dbl)
        n201 = Build Array(w576, w575) -> (w574:dbl[])
        n202 = call-poly <vilib>:"Array To Matrix.vi"("Real 1D Array"=w574) -> ("Real Matrix (Column Vector)"=w573:T1)
        n203 = Transpose Matrix(1:w573) -> (0:w572:T1)
        "Real Matrix 2" <- w572
        n204 = Unbundle(w603) -> ("y"=w582:i32, "x"=w581:i32)
        n205 = Build Array(w582, w581, 1) -> (w579:i32[])
        n206 = call-poly <vilib>:"Array To Matrix.vi"("Real 1D Array"=w579) -> ("Real Matrix (Column Vector)"=w578:T1)
        n207 = Transpose Matrix(1:w578) -> (0:w577:T1)
        "Real Matrix" <- w577
        n208 = call-poly <vilib>:"A x B.vi"("B"=w584, "A"=w577) -> ("A x B"=w592:T1)  [unwired: 1 out]
        "A x B" <- w592
        n209 = call-poly <vilib>:"A x B.vi"("B"=w583, "A"=w572) -> ("A x B"=w587:T1)  [unwired: 1 out]
        "A x B 2" <- w587
        n210 = call-poly <vilib>:"Matrix To Array.vi"("Real Matrix"=w592) -> ("Real 2D Array"=w591:dbl[][])
        n211 = call-poly <vilib>:"Matrix To Array.vi"("Real Matrix"=w587) -> ("Real 2D Array"=w589:dbl[][])
        n212 = Reshape Array(w591, 2) -> (w586:dbl[])
        n213 = Reshape Array(w589, 2) -> (w585:dbl[])
        n214 = Build Array (concatenate)(w601, w600, w586, w585) -> (w599:dbl[])
        n215 = case shown="True" w593 {
          tunnel: [w675 w678] -> w620
          tunnel: w606 -> [_ w680]
          tunnel: w599 -> [_ w679]
          tunnel: w597 -> [_ w676]
          frame False {
            n216 = call <vilib>:"High Resolution Relative Seconds.vi"() -> ("relative seconds"=w675:dbl)
          }
          frame True {
            n217 = disable-structure shown="Disabled" {
              disable-tunnel: w676 -> [w682 _]
              frame Disabled {
                n218 = case shown="True" "display" {
                  tunnel: w682 -> [_ w683]
                  frame False {
                  }
                  frame True {
                    "Image" <- w683
                  }
                }
              }
              frame Enabled {
              }
            }
            n219 = call <vilib>:"High Resolution Relative Seconds.vi"() -> ("relative seconds"=w678:dbl)
            n220 = Build Array (concatenate)(w678, w679) -> (w677:dbl[])
            n221 = Lossy Enqueue Element(queue=w680, element=w677) -> ()  [unwired: 1 in, 4 out]
          }
        }
        n222 = And(x=w609, y="Track") -> (x .and. y?=w596:bool)
        n223 = case shown="True" w596 {
          tunnel: [w696 w755] -> w618
          tunnel: [w697 w756] -> w617
          tunnel: w634 -> [w687 w820]
          tunnel: w633 -> [w694 w819]
          tunnel: w632 -> [w692 w818]
          tunnel: w582 -> [_ w741]
          tunnel: w581 -> [_ w742]
          tunnel: w576 -> [_ w810]
          tunnel: w575 -> [_ w809]
          tunnel: w631 -> [w690 w803]
          tunnel: w601 -> [_ w801]
          tunnel: w600 -> [_ w800]
          tunnel: [w688 w781] -> w630
          tunnel: [w689 w786] -> w629
          tunnel: [w693 w785] -> w628
          tunnel: [w691 w784] -> w627
          tunnel: w619 -> [_ w761]
          tunnel: w622 -> [w695 w760]
          tunnel: [w695 w759] -> w621
          tunnel: w620 -> [_ w757]
          frame False {
            n224 = event shown="[1] \"Controller\": Mouse Down" {
              selector: _ -> [_ _ _]
              dyn-events: _ -> [_ _ _]
              timeout: 1 -> [_ _ _]
              event "Controller": Mouse Up {
                n225 = event-data() -> ()  [unwired: 1 in, 8 out]
                n226 = local write "x"(0.0) -> ()
                n227 = local write "y"(0.0) -> ()
              }
              event "Controller": Mouse Down {
                n228 = event-data() -> ("Coords"=w724:T11)  [unwired: 1 in, 7 out]
                n229 = property on="Controller" class="Pict"() -> ("Position"=w723:T12, "Bounds"=w718:T13)  [unwired: 2 in, 2 out]
                n230 = Unbundle By Name(w724) -> ("Horizontal"=w722:i32, "Vertical"=w720:i32)
                n231 = Unbundle By Name(w718) -> ("Width"=w716:u32, "Height"=w712:u32)
                n232 = Unbundle By Name(w723) -> ("Left"=w721:i32, "Top"=w719:i32)
                n233 = Subtract(x=w720, y=w719) -> (x-y=w713:i32)
                n234 = Subtract(x=w722, y=w721) -> (x-y=w717:i32)
                n235 = Divide(x=w713, y=w712) -> (x/y=w705:dbl)
                n236 = Divide(x=w717, y=w716) -> (x/y=w715:dbl)
                n237 = Subtract(x=w705, y=0.5) -> (x-y=w708:dbl)
                n238 = Subtract(x=w715, y=0.5) -> (x-y=w709:dbl)
                n239 = Multiply(x=w709, y=-5.0) -> (x*y=→"x":dbl)
                n240 = Multiply(x=w708, y=-5.0) -> (x*y=→"y":dbl)
              }
              event Timeout {
                n241 = event-data() -> ()  [unwired: 1 in, 3 out]
              }
            }
            n242 = Get Queue Status(queue=w687) -> (queue out=w686:refnum<queue>, max queue size=w685:i32)  [unwired: 2 in, 6 out]
            n243 = for "For循环" {
              N: w685 -> [_]
              tunnel: w686 -> [w701]
              tunnel: [w700] -> w688
              n244 = Lossy Enqueue Element(queue=w701, element=0.0) -> (queue out=w700:refnum<queue>)  [unwired: 1 in, 3 out]
            }
            n245 = Flush Queue(queue=w694) -> (queue out=w693:refnum<queue>)  [unwired: 1 in, 2 out]
            n246 = Flush Queue(queue=w692) -> (queue out=w691:refnum<queue>)  [unwired: 1 in, 2 out]
            n247 = Flush Queue(queue=w690) -> (queue out=w689:refnum<queue>)  [unwired: 1 in, 2 out]
            n248 = local read "y"() -> (w697:dbl)
            n249 = local read "x"() -> (w696:dbl)
          }
          frame True {
            w746 = 0
            w753 = 23
            w766 = 0.0
            w775 = 2
            w779 = TRUE
            w791 = 1.0
            n250 = local read "Target Y"() -> (w743:i32)
            n251 = Subtract(x=w742, y=w743) -> (x-y=w737:i32)
            n252 = Absolute Value(x=w737) -> (abs(x)=w736:i32)
            n253 = Bundle("Target X"="Target X", "Target Y"="Target Y") -> (w762:cluster{"Target X":i32, "Target Y":i32})  [unwired: 1 in]
            n254 = Greater?(x=w736, y=w753) -> (0:w751:bool)
            n255 = local read "Target X"() -> (w740:i32)
            n256 = Get Queue Status(queue=w820, return elements? (F)=w779) -> (queue out=w782:refnum<queue>, elements=w770:dbl[])  [unwired: 1 in, 6 out]
            n257 = Subtract(x=w741, y=w740) -> (x-y=w735:i32)
            n258 = Get Queue Status(queue=w819) -> (queue out=w814:refnum<queue>, max queue size=w773:i32, # elements in queue=w815:i32)  [unwired: 2 in, 5 out]
            n259 = Equal?(x=w815, y=0) -> (x = y?=w816:bool)
            n260 = Absolute Value(x=w735) -> (abs(x)=w734:i32)
            n261 = Quotient & Remainder(x=w773, y=2) -> (floor(x/y)=w771:i32)  [unwired: 1 out]
            n262 = case shown="True" w816 {
              tunnel: w814 -> [w897 w900]
              tunnel: w741 -> [w896 w901]
              tunnel: w771 -> [_ w902]
              tunnel: [w893 w899] -> w813
              tunnel: w742 -> [w895 w898]
              frame False {
                n263 = Lossy Enqueue Element(queue=w897, element=w896) -> (queue out=w894:refnum<queue>)  [unwired: 1 in, 3 out]
                n264 = Lossy Enqueue Element(queue=w894, element=w895) -> (queue out=w893:refnum<queue>)  [unwired: 1 in, 3 out]
              }
              frame True {
                n265 = for "For循环" {
                  N: w902 -> [_]
                  tunnel: w901 -> [w907]
                  tunnel: w900 -> [w906]
                  tunnel: [w903] -> w899
                  tunnel: w898 -> [w904]
                  n266 = Lossy Enqueue Element(queue=w906, element=w907) -> (queue out=w905:refnum<queue>)  [unwired: 1 in, 3 out]
                  n267 = Lossy Enqueue Element(queue=w905, element=w904) -> (queue out=w903:refnum<queue>)  [unwired: 1 in, 3 out]
                }
              }
            }
            n268 = Get Queue Status(queue=w813, return elements? (F)=w779) -> (queue out=w785:refnum<queue>, elements=w780:i32[])  [unwired: 1 in, 6 out]
            n269 = Greater?(x=w734, y=w753) -> (0:w752:bool)
            n270 = Or(x=w751, y=w752) -> (x .or. y?=w750:bool)
            n271 = Get Queue Status(queue=w818) -> (queue out=w807:refnum<queue>, max queue size=w776:i32, # elements in queue=w811:i32)  [unwired: 2 in, 5 out]
            n272 = Equal?(x=w811, y=0) -> (x = y?=w808:bool)
            n273 = Select(t=1, s=w750, f=w746) -> (s? t:f=w748:i32)
            n274 = Quotient & Remainder(x=w776, y=w775) -> (floor(x/y)=w774:i32)  [unwired: 1 out]
            n275 = case shown="True" w808 {
              tunnel: w807 -> [w882 w885]
              tunnel: w810 -> [w881 w886]
              tunnel: w774 -> [_ w887]
              tunnel: [w878 w884] -> w806
              tunnel: w809 -> [w880 w883]
              frame False {
                n276 = Lossy Enqueue Element(queue=w882, element=w881) -> (queue out=w879:refnum<queue>)  [unwired: 1 in, 3 out]
                n277 = Lossy Enqueue Element(queue=w879, element=w880) -> (queue out=w878:refnum<queue>)  [unwired: 1 in, 3 out]
              }
              frame True {
                n278 = for "For循环" {
                  N: w887 -> [_]
                  tunnel: w886 -> [w892]
                  tunnel: w885 -> [w891]
                  tunnel: [w889] -> w884
                  tunnel: w883 -> [w888]
                  n279 = Lossy Enqueue Element(queue=w891, element=w892) -> (queue out=w890:refnum<queue>)  [unwired: 1 in, 3 out]
                  n280 = Lossy Enqueue Element(queue=w890, element=w888) -> (queue out=w889:refnum<queue>)  [unwired: 1 in, 3 out]
                }
              }
            }
            n281 = Get Queue Status(queue=w806, return elements? (F)=w779) -> (queue out=w784:refnum<queue>, elements=w768:dbl[])  [unwired: 1 in, 6 out]
            n282 = local read "m(length of kernel)"() -> (w798:i32)
            n283 = local read "length of fish_history"() -> (w796:i32)
            n284 = feedback #6(w746) -> (w732:i32)
            n285 = Divide(x=1.0, y=30.0) -> (x/y=w793:dbl)
            n286 = expression code="atan(x)"(-0.043) -> (w792:dbl)
            n287 = Get Queue Status(queue=w803) -> (queue out=w802:refnum<queue>, max queue size=w778:i32, # elements in queue=w804:i32)  [unwired: 2 in, 5 out]
            n288 = Quotient & Remainder(x=w778, y=w775) -> (floor(x/y)=w777:i32)  [unwired: 1 out]
            n289 = Equal?(x=w804, y=0) -> (x = y?=w758:bool)
            n290 = case shown="True" w758 {
              tunnel: w802 -> [w867 w870]
              tunnel: w801 -> [w866 w871]
              tunnel: w777 -> [_ w872]
              tunnel: [w863 w869] -> w799
              tunnel: w800 -> [w865 w868]
              frame False {
                n291 = Lossy Enqueue Element(queue=w867, element=w866) -> (queue out=w864:refnum<queue>)  [unwired: 1 in, 3 out]
                n292 = Lossy Enqueue Element(queue=w864, element=w865) -> (queue out=w863:refnum<queue>)  [unwired: 1 in, 3 out]
              }
              frame True {
                n293 = for "For循环" {
                  N: w872 -> [_]
                  tunnel: w871 -> [w877]
                  tunnel: w870 -> [w876]
                  tunnel: [w873] -> w869
                  tunnel: w868 -> [w874]
                  n294 = Lossy Enqueue Element(queue=w876, element=w877) -> (queue out=w875:refnum<queue>)  [unwired: 1 in, 3 out]
                  n295 = Lossy Enqueue Element(queue=w875, element=w874) -> (queue out=w873:refnum<queue>)  [unwired: 1 in, 3 out]
                }
              }
            }
            n296 = Get Queue Status(queue=w799, return elements? (F)=w779) -> (queue out=w786:refnum<queue>, elements=w769:i32[])  [unwired: 1 in, 6 out]
            n297 = Max & Min(x=w734, y=w736) -> (max(x,y)=w745:i32)  [unwired: 1 out]
            n298 = Divide(x=w791, y=10000.0) -> (x/y=w788:dbl)
            n299 = Divide(x=w791, y=12800.0) -> (x/y=w787:dbl)
            n300 = feedback #7(w746) -> (w738:i32)
            n301 = case shown="True" "count" {
              tunnel: [w821 w823] -> w739
              tunnel: w738 -> [_ w822]
              tunnel: w732 -> [_ w823]
              tunnel: [w821 w822] -> w731
              frame False {
                w821 = 0
                "out of FOV 2" <- w821
                "max distance 2" <- w821
              }
              frame True {
                "out of FOV" <- w823
                "max distance" <- w822
              }
            }
            n302 = Add(x=w739, y=w748) -> (x+y=w747:i32)
            n303 = feedback-in #6(w747) -> ()
            n304 = Max & Min(x=w745, y=w731) -> (max(x,y)=w744:i32)  [unwired: 1 out]
            n305 = feedback-in #7(w744) -> ()
            n306 = Bundle(w766, w766) -> (w765:cluster{dbl, dbl})  [unwired: 1 in]
            n307 = dll-call lib="F:/TrackingUsingOpenCV3_with_bkg_subtr_and_pred_and_temp_matching_nodisplay - 210309/MPC_dll_4_vs17_cv3_4/x64/Release/MPC_dll_4_vs17_cv3_4.dll" fn="?MPC_dll@@YAHHHHNNNHNNNNNPEAV?$Point_@H@cv@@PEANPEAH21PEAV?$Point_@N@2@@Z"("m"=w798, "predict_length"=6 ("predict length"), "fish_history_length"=w796, "gammaX"="gamma", "gammaY"="gamma", "max_command"=10.0, "shift_head2yolk"=18, "scale_x"=w793, "scale_y"=w793, "theta"=w792, "scale_x2"=w788, "scale_y2"=w787, "dst_fish_position"=w762, "command_history_array"=w770, "position_history_array"=w769, "fish_tr_history_c_array"=w780, "fish_direction_history_c_array"=w768, "c0"=w765) -> ("return type"=w730:i32, "c0"=w767:cluster{dbl, dbl})  [unwired: 20 in, 2 out]
            n308 = Equal To 0?(x=w730) -> (x = 0?=w728:bool)
            n309 = Not(x=w728) -> (.not. x?=w729:bool)
            n310 = case shown="False" w729 {
              tunnel: w761 -> [w850 w862]
              tunnel: w760 -> [w849 w861]
              tunnel: [w849 w860] -> w759
              tunnel: w757 -> [w851 w859]
              frame False {
                w839 = -inf
                n311 = local read "time loading a frame"() -> (w842:dbl)
                n312 = local read "TimeDelay"() -> (w844:dbl)
                n313 = call <vilib>:"High Resolution Relative Seconds.vi"() -> ("relative seconds"=w852:dbl)
                n314 = Not(x="reset 2") -> (.not. x?=w828:bool)
                n315 = Boolean To (0,1)(Boolean=w828) -> (0, 1=w827:i16)
                n316 = Subtract(x=w852, y=w850) -> (x-y=w829:dbl)
                n317 = Subtract(x=w851, y=w850) -> (x-y=w846:dbl)
                n318 = feedback #8(w839) -> (w848:dbl)
                n319 = feedback #9(w839) -> (w845:dbl)
                n320 = feedback #10(w839) -> (w847:dbl)
                n321 = Max & Min(x=w829, y=w848) -> (max(x,y)=w838:dbl)  [unwired: 1 out]
                "max time1 detection+command" <- w838
                n322 = feedback-in #8(w838) -> ()
                n323 = Max & Min(x=w844, y=w845) -> (max(x,y)=w841:dbl)  [unwired: 1 out]
                "max time3 total" <- w841
                n324 = feedback-in #9(w841) -> ()
                n325 = Max & Min(x=w846, y=w847) -> (max(x,y)=w826:dbl)  [unwired: 1 out]
                "max time2 detection" <- w826
                n326 = Multiply(x=w826, y=w827) -> (x*y=w825:dbl)
                n327 = feedback-in #10(w825) -> ()
                n328 = Greater?(x=w829, y=0.003) -> (0:w836:bool)
                n329 = feedback #11(w839) -> (w843:dbl)
                n330 = Select(t=1, s=w836, f=0) -> (s? t:f=w833:i32)
                n331 = Max & Min(x=w842, y=w843) -> (max(x,y)=w840:dbl)  [unwired: 1 out]
                "max time4 image and position loading" <- w840
                n332 = feedback-in #11(w840) -> ()
                n333 = feedback #12(0) -> (w832:i32)
                n334 = Add(x=w833, y=w832) -> (x+y=w831:i32)
                "#timeout1" <- w831
                n335 = feedback-in #12(w831) -> ()
              }
              frame True {
                n336 = call <vilib>:"High Resolution Relative Seconds.vi"() -> ("relative seconds"=w858:dbl)
                n337 = local read "TimeDelay"() -> (w856:dbl)
                n338 = local read "time loading a frame"() -> (w853:dbl)
                n339 = Subtract(x=w858, y=w862) -> (x-y=w857:dbl)
                n340 = Subtract(x=w859, y=w862) -> (x-y=w855:dbl)
                n341 = Format Into String(initial string=w861, w857, w855, w856, w853, "\r") -> (resulting string=w860:refnum<file>)  [unwired: 2 in, 1 out]
              }
            }
            n342 = Unbundle(w767) -> (w755:dbl, w756:dbl)
            n343 = Lossy Enqueue Element(queue=w782, element=w755) -> (queue out=w783:refnum<queue>)  [unwired: 1 in, 3 out]
            n344 = Lossy Enqueue Element(queue=w783, element=w756) -> (queue out=w781:refnum<queue>)  [unwired: 1 in, 3 out]
          }
        }
      }
      frame #3 {
      }
      frame #4 {
        n345 = Negate(x=w920) -> (-x=w919:dbl)
        "电压2" <- w919
        n346 = call-poly <vilib>:"DAQmx Write.vi"("task/channels in"=w923, "data"=w921) -> ("task out"=w924:refnum<k21>)  [unwired: 11 in, 2 out]
        n347 = call-poly <vilib>:"DAQmx Write.vi"("task/channels in"=w922, "data"=w919) -> ("task out"=w925:refnum<k21>)  [unwired: 11 in, 2 out]
        "电压1" <- w921
      }
      frame #5 {
        n348 = call <vilib>:"High Resolution Relative Seconds.vi"() -> ("relative seconds"=w935:dbl)
      }
    }
    n349 = flat-sequence {
      tunnel: w312 -> [w949]
      tunnel: [w947] -> w419
      frame #0 {
        n350 = Unbundle By Name(w949) -> ("status"=w950:bool)
        n351 = local read "Stopped"() -> (w948:bool)
        n352 = Compound Arithmetic op=OR(w950, "Stop", w948) -> (w947:bool)
        n353 = local write "Stopped"(w947) -> ()
      }
    }
    n354 = feedback-in #13(w419) -> ()
    n355 = feedback #13() -> (w418:bool)  [unwired: 1 in]
    n356 = node-c288() -> ()  [unwired: 1 in, 1 out]
  }
  n357 = Close File(refnum=w30) -> ()  [unwired: 1 in, 2 out]
  n358 = call-poly <vilib>:"DAQmx Write.vi"("task/channels in"=w83, "data"=0.0) -> ("task out"=w81:refnum<k21>)  [unwired: 11 in, 2 out]
  n359 = call <vilib>:"DAQmx Stop Task.vi"("task/channels in"=w81) -> ("task out"=w77:refnum<k21>)  [unwired: 13 in, 1 out]
  n360 = call-poly <vilib>:"DAQmx Write.vi"("task/channels in"=w82, "data"=0.0) -> ("task out"=w79:refnum<k21>)  [unwired: 11 in, 2 out]
  n361 = call <vilib>:"DAQmx Stop Task.vi"("task/channels in"=w79) -> ("task out"=w76:refnum<k21>)  [unwired: 13 in, 1 out]
  n362 = call <vilib>:"DAQmx Clear Task.vi"("task in"=w77) -> ()  [unwired: 14 in, 1 out]
  n363 = call <vilib>:"DAQmx Clear Task.vi"("task in"=w76) -> ()  [unwired: 14 in, 1 out]
  n364 = node-c288(w16) -> ()  [unwired: 1 out]
  n365 = Release Queue(queue=w37) -> ()  [unwired: 2 in, 3 out]
  n366 = Release Queue(queue=w36) -> ()  [unwired: 2 in, 3 out]
  n367 = Release Queue(queue=w35) -> ()  [unwired: 2 in, 3 out]
  n368 = Release Queue(queue=w34) -> ()  [unwired: 2 in, 3 out]
  n369 = call <userlib>:"DAQNavi Stop Task.vi"("task in"=w58) -> ("task out"=w60:i32)  [unwired: 1 in, 1 out]
  n370 = Merge Errors(w116, w115) -> (w117:errorcluster)
  n371 = call <userlib>:"DAQNavi Stop Task.vi"("task in"=w57) -> ("task out"=w59:i32)  [unwired: 1 in, 1 out]
  n372 = flat-sequence {
    tunnel: w117 -> [w953]
    tunnel: [w953] -> w124
    tunnel: w123 -> [w954]
    tunnel: w9 -> [_]
    frame #0 {
      n373 = local write "Initialized"(FALSE ("Module Enabled")) -> ()
      n374 = call "IMAQ Dispose"("Image"=w954) -> ()  [unwired: 5 in, 1 out]
    }
  }
  n375 = call <userlib>:"DAQNavi Clear Task.vi"("task in"=w60) -> ()  [unwired: 2 in, 1 out]
  n376 = call <userlib>:"DAQNavi Clear Task.vi"("task in"=w59) -> ()  [unwired: 2 in, 1 out]
  n377 = xnode "关闭FPGA VI引用"("FPGA VI引用输入"=w125, "错误输入"=w124) -> ("错误输出"=w122:errorcluster)
  n378 = call <vilib>:"Simple Error Handler.vi"("error in (no error)"=w122) -> ()  [unwired: 4 in, 5 out]
